vi "Task06.vi"() -> ()   [LabVIEW 2017]
panel:
  out "Waveform Chart":u32(graph)
  in  "stop":bool
  out "Indicator":dbl
  in  "Array":bool[](array[boolean])
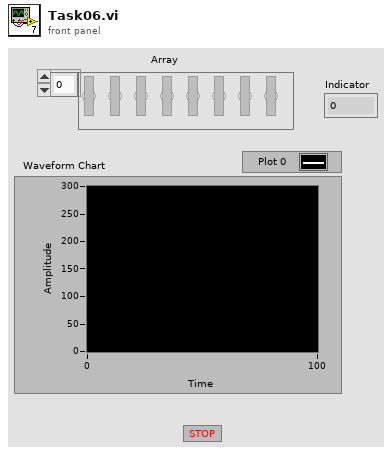
[diagram p1: front panel]
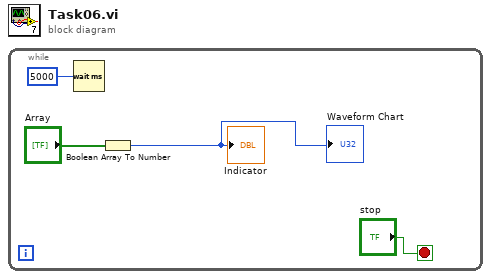
[diagram p0: block diagram]
diagram:
  n1 = while {
    stop <- "stop" stop-if-true
    n2 = Wait (ms)(milliseconds to wait=5000) -> ()  [unwired: 1 out]
    n3 = Boolean Array To Number(Boolean array="Array") -> (number=→"Indicator" →"Waveform Chart":u32)
  }
